vi "Socket.TCP Echo Server.vi"() -> ()   [LabVIEW 2014]
uses:
  Classes/Socket.TCP/Socket.TCP.lvclass
  Classes/Socket.Base/Socket.Base.lvclass/Socket.Base.ctl
  Classes/Socket.TCP/Socket.TCP.lvclass/Socket.TCP.ctl
  Classes/Socket.Base/Accessors/Write timeout.vi
  Classes/Socket.TCP/Accessors/Read remote_address .vi
  Classes/Socket.TCP/Accessors/Read remote_port .vi
panel:
  out "Data From Client":string
  out "error out":errorcluster
  in  "Stop Button":bool
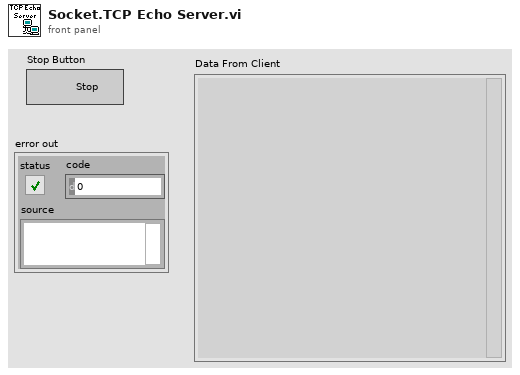
[diagram p1: front panel]
types:
  T1 = enum16{"Standard", "Buffered", "CRLF", "Immediate"}
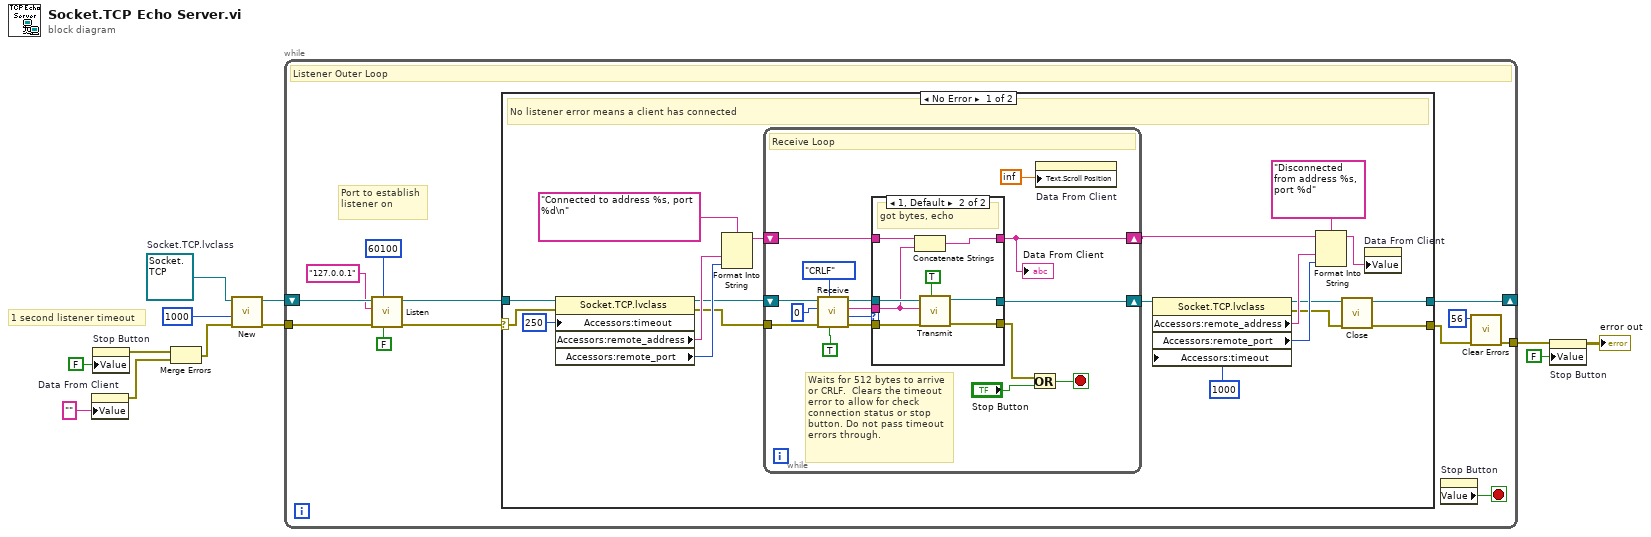
[diagram p0: block diagram]
diagram:
  w12 = refnum<class "Socket.TCP.lvclass"> refnum  # Socket.TCP.lvclass
  # "1 second listener timeout"
  n1 = property on="Data From Client" class="Str"("Value"="") -> (error out=w2:errorcluster)  [unwired: 2 in, 1 out]
  n2 = property on="Stop Button" class="Bool (strict)"("Value"=FALSE ("Stop Button")) -> (error out=w9:errorcluster)  [unwired: 2 in, 1 out]
  n3 = Merge Errors(w9, w2) -> (w8:errorcluster)
  n4 = call-dynamic "New.vi"("error in (no error)"=w8, "timeout"=1000 ("timeout (10000)"), "Socket.TCP in"=w12) -> ("error out"=w6:errorcluster, "Socket.TCP out"=w7:refnum<class "Socket.TCP.lvclass">)  [unwired: 7 in]
  n5 = while {
    tunnel: w6 -> [w23]
    shift-right: [w17] -> _
    shift-left: w7 -> [w24]
    tunnel: [w14] -> w4
    stop <- w13 stop-if-true
    # "Port to establish listener on"
    # "Listener Outer Loop"
    n6 = call "Listen.vi"("clear_timeout_error (f)"=FALSE, "listener_port"=u16 60100, "error in (no error)"=w23, "net_address"="127.0.0.1", "Socket.TCP in"=w24) -> ("error out"=w18:errorcluster, "Socket.TCP out"=w19:refnum<class "Socket.TCP.lvclass">)  [unwired: 5 in]
    n7 = case shown="No Error" w18 {
      selector: w18 -> [w43 w73]
      tunnel: w19 -> [w44 w72]
      tunnel: [w27 w72] -> w17
      tunnel: [w26 w73] -> w15
      frame No Error {
        # "No listener error means a client has connected"
        n8 = property class="Socket.TCP.lvclass"(reference=w44, error in=w43, "Accessors:timeout"=250 ("timeout (10000)")) -> (reference out=w38:refnum<class "Socket.TCP.lvclass">, error out=w37:errorcluster, "Accessors:remote_address "=w40:string, "Accessors:remote_port "=w39:u16)
        n9 = Format Into String(format string="Connected to address %s, port %d\n", w40, w39) -> (resulting string=w36:string)  [unwired: 2 in, 1 out]
        n10 = while {
          tunnel: w37 -> [w59]
          shift-right: [w47] -> w32
          shift-left: w36 -> [w52]
          shift-right: [w46] -> w35
          shift-left: w38 -> [w60]
          stop <- w48 stop-if-true
          # "Waits for 512 bytes to arrive or CRLF.  Clears the timeout error to allow for check connection status or stop button. Do not pass timeout errors through."
          # "Receive Loop"
          n11 = call-dynamic "Receive.vi"("clear_timeout_error (f)"=TRUE, "mode (standard)"=T1."CRLF", "error in (no error)"=w59, "bufsize (0)"=u32 0, "Socket.TCP in"=w60) -> ("error out"=w55:errorcluster, "bytes_read"=w56:i32, "data_out"=w54:string, "Socket.TCP out"=w53:refnum<class "Socket.TCP.lvclass">)  [unwired: 3 in]
          n12 = case shown="1, Default" w56 {
            tunnel: w55 -> [w61 w71]
            tunnel: w54 -> [_ w68]
            tunnel: w53 -> [w62 w70]
            tunnel: w52 -> [w63 w69]
            tunnel: [w63 w67] -> w47
            tunnel: [w62 w66] -> w46
            tunnel: [w61 w65] -> w50
            frame 0 {
              # "0 bytes likely timeout"
            }
            frame 1, Default {
              # "got bytes, echo"
              n13 = Concatenate Strings(w69, w68) -> (w67:string)
              n14 = call-dynamic "Transmit.vi"("packet? (f)"=TRUE, "error in (no error)"=w71, "data"=w68, "Socket.TCP in"=w70) -> ("error out"=w65:errorcluster, "Socket.TCP out"=w66:refnum<class "Socket.TCP.lvclass">)  [unwired: 5 in, 1 out]
            }
          }
          "Data From Client" <- w47
          n15 = Or(x=w50, y="Stop Button") -> (x .or. y?=w48:bool)
          n16 = property on="Data From Client" class="Str"("Text.Scroll Position"=inf) -> ()  [unwired: 2 in, 2 out]
        }
        n17 = property class="Socket.TCP.lvclass"(reference=w35, "Accessors:timeout"=1000 ("timeout")) -> (reference out=w29:refnum<class "Socket.TCP.lvclass">, error out=w28:errorcluster, "Accessors:remote_address "=w31:string, "Accessors:remote_port "=w30:u16)  [unwired: 1 in]
        n18 = Format Into String(format string="Disconnected from address %s, port %d", initial string=w32, w31, w30) -> (resulting string=w25:string)  [unwired: 1 in, 1 out]
        n19 = call-dynamic "Close.vi"("error in (no error)"=w28, "Socket.TCP in"=w29) -> ("error out"=w26:errorcluster, "Socket.TCP out"=w27:refnum<class "Socket.TCP.lvclass">)  [unwired: 8 in]
        n20 = property on="Data From Client" class="Str"("Value"=w25) -> ()  [unwired: 2 in, 2 out]
      }
      frame Error {
        # "Listener error means no client has connected yet"
      }
    }
    n21 = property on="Stop Button" class="Bool (strict)"() -> ("Value"=w13:bool)  [unwired: 2 in, 2 out]
    n22 = call <vilib>:"Clear Errors.vi"("error in (no error)"=w15, "specific error code to clear (0: all)"=56) -> ("error out"=w14:errorcluster)  [unwired: 4 in, 1 out]
  }
  n23 = property on="Stop Button" class="Bool (strict)"(error in=w4, "Value"=FALSE ("Stop Button")) -> (error out=→"error out":errorcluster)  [unwired: 1 in, 1 out]
